vi "Run Child.vi"(8 "error in (no error)":errorcluster, 9 "Working Path":path, 10 "UI":refnum<class "UI.lvclass">, 11 "Upgrade in":refnum<class "Upgrade.lvclass">) -> (0 "error out":errorcluster, 3 "Upgrade out":refnum<class "Upgrade.lvclass">)   [LabVIEW 2020, in "Upgrade.lvlib" / "Upgrade.lvclass"]
uses:
  Upgrade.lvclass
  build/ppl/neg-pkg.lvlibp/neg-pkg/UI/UI.lvclass
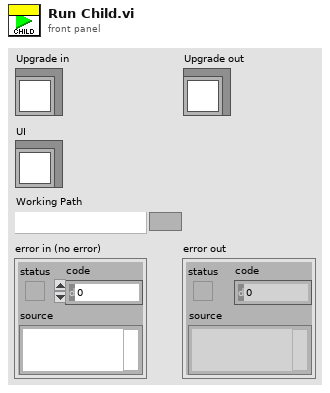
[diagram p1: front panel]
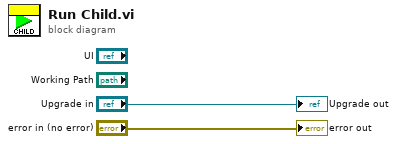
[diagram p0: block diagram]
diagram:
  "error out" <- "error in (no error)"
  "Upgrade out" <- "Upgrade in"
